vi "Main.vi"(11 "Module Admin":refnum<class "Delacor_lib_QMH_Cloneable Module Admin.lvclass">) -> ()   [LabVIEW 2020, in "My Cloneable Module.lvlib"]
doc: "This template is based off of the Queued Message Handler design pattern and the Queued Message Handler project template that ships with LabVIEW.\n\nThe main difference is that the queue is private to this module and communication between modules is performed via Broadcast and Request events.\n\nRequest events are wrapped in public API methods and are handled in the Event Handling Loop (EHL) of this VI. Any module can register for Broadcast events sent by this module. The EHL generates messages based on user interface actions.\n\nThe Message Handling Loop (MHL) processes messages generated by the EHL, or by other messages. The messages are string values, so new messages can be added easily to the Message Cases case structure in the MHL. Each message cluster can also provide an optional value for Message Data, which is a variant that can be converted to whatever message-specific data is required.\n_____\nBased on Delacor QMH Project Template 5.0.0.82."
uses:
  My Cloneable Module.lvlib
  <vilib>/Delacor/Delacor QMH/Libraries/Cloneable Module Admin_class/Delacor_lib_QMH_Cloneable Module Admin.lvclass
  C:/Program Files (x86)/National Instruments/LabVIEW 2020/vi.lib/Delacor/Delacor QMH/Libraries/Module Admin_class/Delacor_lib_QMH_Module Admin.lvclass
  Module Data--cluster.ctl
  Do Something Argument--cluster.ctl
  <vilib>/Delacor/Delacor QMH/Libraries/Cloneable Module Admin_class/Delacor_lib_QMH_Cloneable Module Admin.lvclass/Delacor_lib_QMH_Cloneable Module Admin.ctl
  <vilib>/Delacor/Delacor QMH/Libraries/Message Queue_class/Delacor_lib_QMH_Message Queue.lvclass/Delacor_lib_QMH_Message Queue.ctl
  Do Something Else Argument--cluster.ctl
  Do Something Else and Wait for Reply Argument--cluster.ctl
  Do Something Else and Wait (Reply Payload)--cluster.ctl
  Stop Argument--cluster.ctl
  <vilib>/Delacor/Delacor QMH/Libraries/Module Admin_class/Delacor_lib_QMH_Module Admin.lvclass/Delacor_lib_QMH_Module Admin.ctl
  <vilib>/Utility/miscctls.llb/LVPointTypeDef.ctl
  <vilib>/Delacor/Delacor QMH/Libraries/Message Queue_class/Delacor_lib_QMH_Enqueue Message (Single).vi
  <vilib>/Delacor/Delacor QMH/Libraries/Cloneable Module Admin_class/Delacor_lib_QMH_Get Module ID.vi
  <vilib>/Delacor/Delacor QMH/Libraries/Module Admin_class/Delacor_lib_QMH_Get External Launch.vi
  <vilib>/Utility/error.llb/Error Cluster From Error Code.vi
  <vilib>/ErrorRing/Error Ring.xnode
  <vilib>/Delacor/Delacor QMH/Libraries/Message Queue_class/Delacor_lib_QMH_Message Queue.lvclass
panel:
  in  "Simulate MHL Error":bool
  in  "Simulate EHL Error":bool
  out "error out":errorcluster
  out "X":dbl
  out "Status":string
  in  "Do Something Else <Replace Me>":bool
  in  "Do Something <Replace Me>":bool
  # "These controls have associated \"Value Changed\" events configured in the Event Structure on the diagram.\n\nReplace them (and reconfigure the Event Structure) with the controls you need for your application. \n\nOther QMH Modules communicate with this Module via its Public API (wrappers for its Request Events).\n\nThis Module communicates with other Modules via its Broadcast Events.\nAny module that wants to get these messages, just registers for this module's Broadcast events."
  # "This template is for the Delacor Modified Queued Message Handler design pattern.\n\nSee the block diagram for more information on how to use this template."
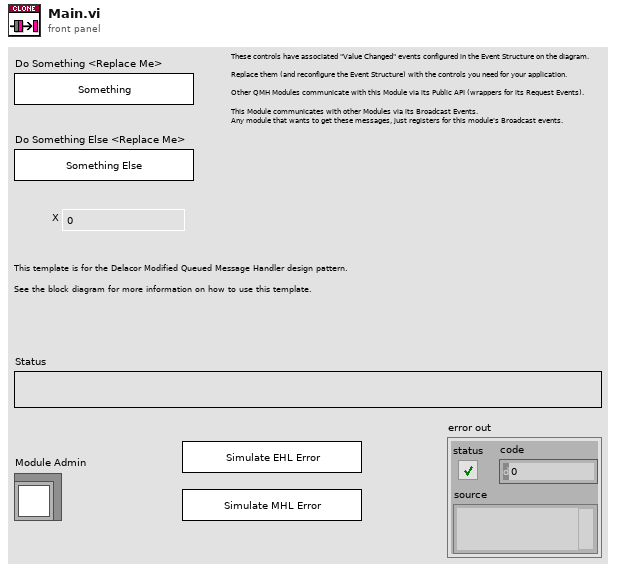
[diagram p1: front panel]
types:
  T1 = typedef "My Cloneable Module.lvlib/Request Events--cluster.ctl" = cluster{"Stop Module":refnum<user-event>, "Do Something":refnum<user-event>, "Do Something Else":refnum<user-event>, "Do Something Else and Wait for Reply":refnum<user-event>, "Show Panel":refnum<user-event>, "Hide Panel":refnum<user-event>, "Show Diagram":refnum<user-event>, "Get Module Execution Status":refnum<user-event>}
  T2 = typedef "My Cloneable Module.lvlib/Module Data--cluster.ctl" = cluster{"Status":string}
  T3 = typedef "My Cloneable Module.lvlib/Do Something Argument--cluster.ctl" = cluster{"Module ID":i32, "Do Something Msg":string}
  T4 = typedef "My Cloneable Module.lvlib/Do Something Else Argument--cluster.ctl" = cluster{"Module ID":i32, "Do Something Else Msg":string, "X":dbl}
  T5 = typedef "My Cloneable Module.lvlib/Do Something Else and Wait for Reply Argument--cluster.ctl" = cluster{"Module ID":i32, "Do Something Else Msg":string, "X":dbl, "Wait Notifier":refnum<notifier>, "wait for reply":bool}
  T6 = enum32{"invalid lock state", "Not Locked", "Locked (No Password)", "Password-protected"}
  T7 = typedef "My Cloneable Module.lvlib/Stop Argument--cluster.ctl" = cluster{"Module ID":i32, "Origin":string, "Exit via Stop Module Req?":bool, "Wait for Module to stop?":bool}
  T8 = typedef "LVPointTypeDef.ctl" = cluster{"Horizontal":i16, "Vertical":i16}
  T9 = enum32{"Invalid", "Standard", "Closed", "Hidden", "Minimized", "Maximized"}
  T10 = typedef "My Cloneable Module.lvlib/Do Something Else and Wait (Reply Payload)--cluster.ctl" = cluster{"Value":dbl, "error":errorcluster}
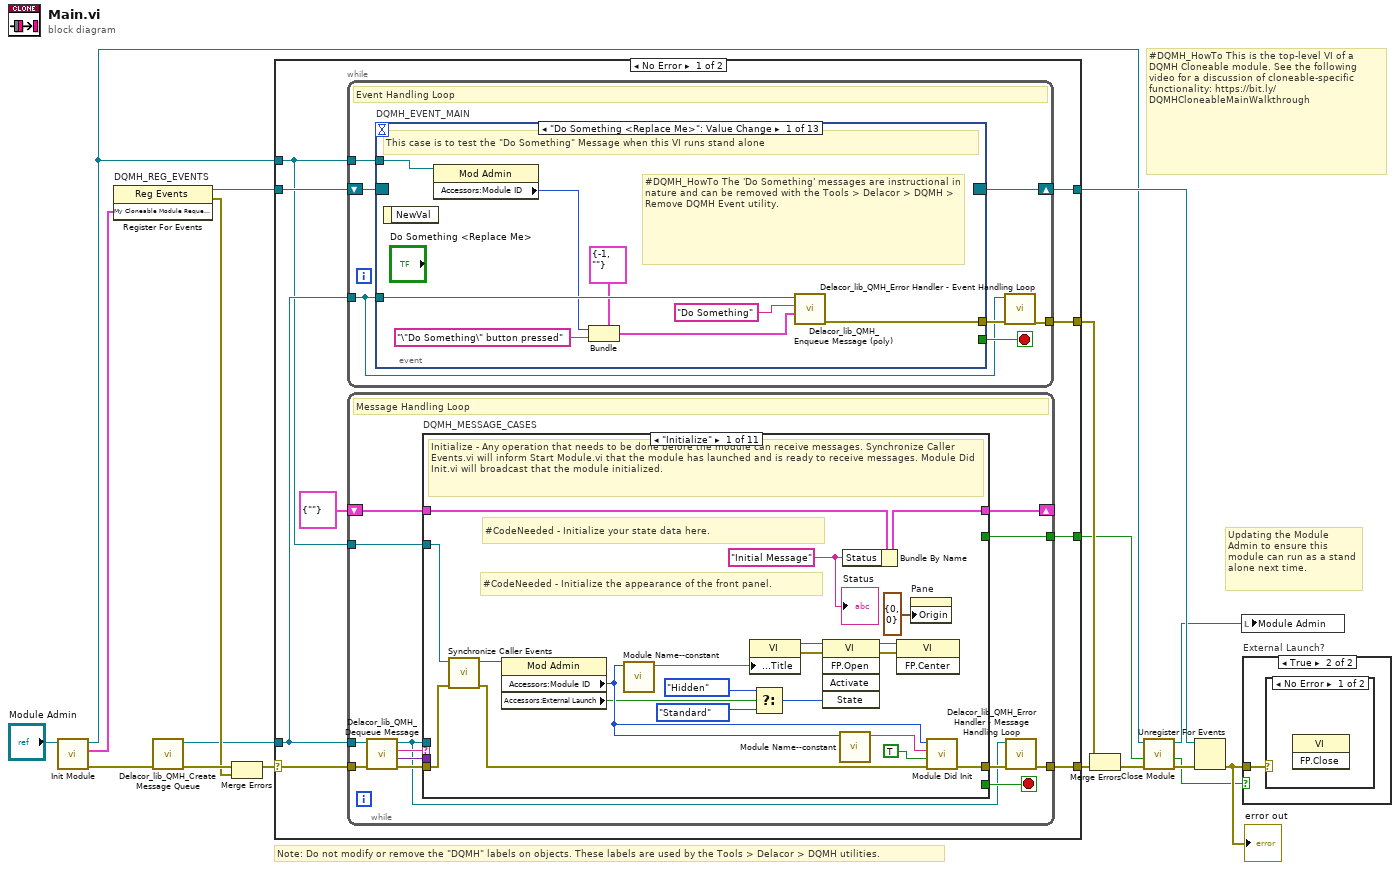
[diagram p0: block diagram]
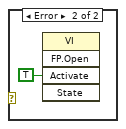
[diagram p3: hidden frame]
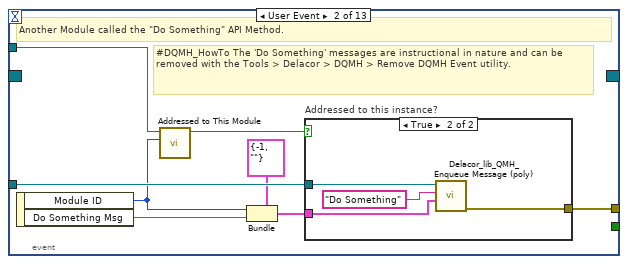
[diagram p4: hidden frame]
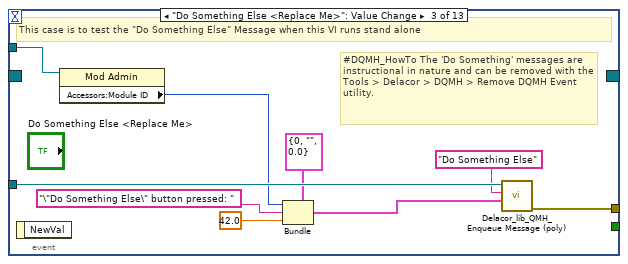
[diagram p6: hidden frame]
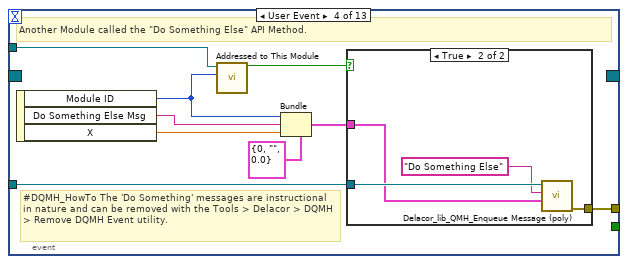
[diagram p7: hidden frame]
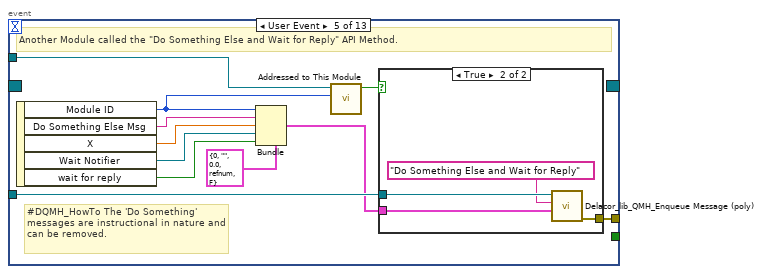
[diagram p9: hidden frame]
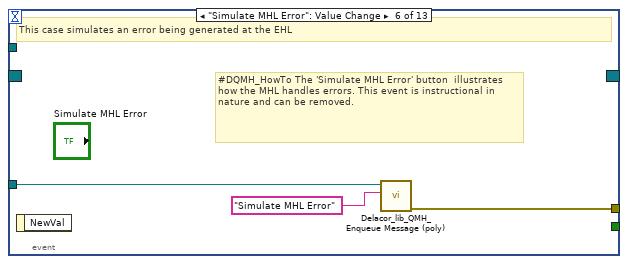
[diagram p11: hidden frame]
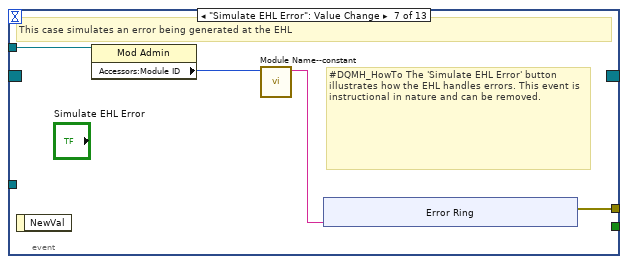
[diagram p12: hidden frame]
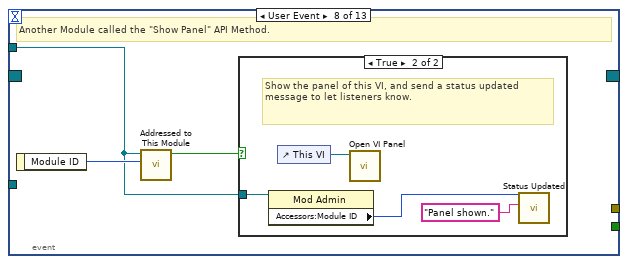
[diagram p13: hidden frame]
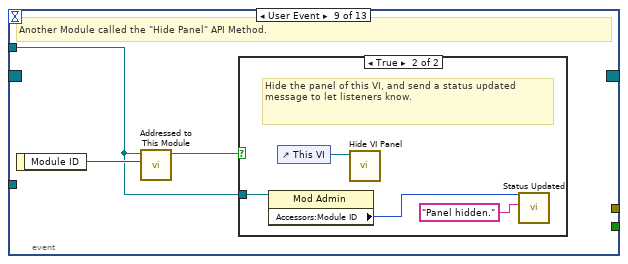
[diagram p15: hidden frame]
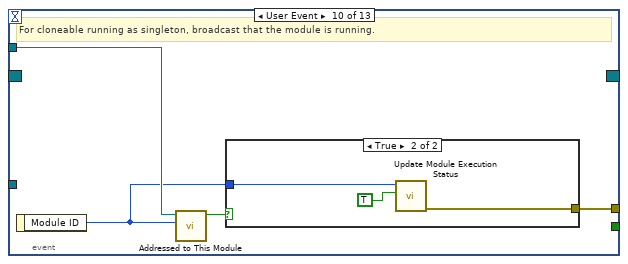
[diagram p17: hidden frame]
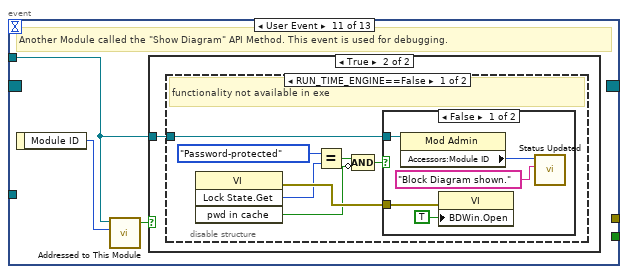
[diagram p19: hidden frame]
diagram:
  # "#DQMH_HowTo This is the top-level VI of a DQMH Cloneable module. See the following video for a discussion of cloneable-specific functionality: https://bit.ly/DQMHCloneableMainWalkthrough"
  # "Note: Do not modify or remove the \"DQMH\" labels on objects. These labels are used by the Tools > Delacor > DQMH utilities."
  # "Updating the Module Admin to ensure this module can run as a stand alone next time."
  n1 = call "Init Module.vi"("Cloneable Module Admin in"="Module Admin") -> ("error out"=w15:errorcluster, "My Cloneable Module Request Events"=w7:T1, "Cloneable Module Admin out"=w4:refnum<class "Delacor_lib_QMH_Cloneable Module Admin.lvclass">)  [unwired: 8 in]
  n2 = register-events "DQMH_REG_EVENTS"(w7) -> (reference out=w8:refnum<event-registration>, error out=w10:errorcluster)  [unwired: 2 in]
  n3 = call <vilib>:"Delacor_lib_QMH_Create Message Queue.vi"("error in (no error)"=w15) -> ("error out"=w12:errorcluster, "Message Queue"=w6:refnum<class "Delacor_lib_QMH_Message Queue.lvclass">)  [unwired: 9 in]
  n4 = Merge Errors(w12, w10) -> (w11:errorcluster)
  n5 = case shown="No Error" w11 {
    selector: w11 -> [w25 w335]
    tunnel: [w27 w334] -> w16
    tunnel: [w24 w342] -> w9
    tunnel: w8 -> [w22 w342]
    tunnel: w6 -> [w21 w333]
    tunnel: [w26 _] -> w17
    tunnel: w4 -> [w20 w338]
    tunnel: [w19 _] -> w2
    frame No Error {
      n6 = while {
        tunnel: w21 -> [w28]
        shift-right: [w31] -> w24
        shift-left: w22 -> [w32]
        tunnel: [w33] -> w26
        tunnel: w20 -> [w29]
        stop <- w30 stop-if-true
        # "Event Handling Loop"
        n7 = event "DQMH_EVENT_MAIN" shown="[0] \"Do Something <Replace Me>\": Value Change" {
          selector: w32 -> [_ _ _ _ _ _ _ _ _ _ _ _ _]
          dyn-events: [_ _ _ _ _ _ _ _ _ _ _ _ _] -> w31
          timeout: _ -> [_ _ _ _ _ _ _ _ _ _ _ _ _]
          tunnel: [_ _ _ _ _ _ _ _ _ _ _ w146 _] -> w30
          tunnel: w28 -> [w41 w49 w62 w71 w86 w93 _ _ _ _ _ w149 w165]
          tunnel: [w42 w50 w63 w72 w87 w94 w98 _ _ w123 _ w150 w168] -> w34
          tunnel: w29 -> [w37 w47 w56 w69 w84 _ w97 w106 w113 w121 w127 w148 w166]
          event "Do Something <Replace Me>": Value Change {
            # "#DQMH_HowTo The 'Do Something' messages are instructional in nature and can be removed with the Tools > Delacor > DQMH > Remove DQMH Event utility."
            # "This case is to test the \"Do Something\" Message when this VI runs stand alone"
            n8 = event-data() -> ()  [unwired: 1 in, 1 out]
            n9 = property class="Mod Admin"(reference=w37) -> ("Accessors:Module ID"=w36:i32)  [unwired: 1 in, 2 out]
            n10 = Bundle(cluster=T3 {"Module ID"=-1, "Do Something Msg"=""} ("Do Something Argument"), "Module ID"=w36, "Do Something Msg"="\"Do Something\" button pressed" ("\"Do Something\" button pressed")) -> (w39:T3)
            n11 = call-poly <vilib>:"Delacor_lib_QMH_Enqueue Message (poly).vi"("Message Data"=w39, "Message"="Do Something", "Message Queue in"=w41) -> ("error out"=w42:errorcluster)  [unwired: 7 in, 1 out]
          }
          event User Event {
            # "#DQMH_HowTo The 'Do Something' messages are instructional in nature and can be removed with the Tools > Delacor > DQMH > Remove DQMH Event utility."
            # "Another Module called the \"Do Something\" API Method."
            n12 = event-data() -> ("Module ID"=w44:i32, "Do Something Msg"=w43:string)  [unwired: 1 in]
            n13 = call "Addressed to This Module.vi"("Module ID from Argument"=w44, "Module Admin"=w47) -> ("Addressed to this instance?"=w48:bool)  [unwired: 8 in, 1 out]
            n14 = Bundle(cluster=T3 {"Module ID"=-1, "Do Something Msg"=""} ("Do Something Argument"), "Module ID"=w44, "Do Something Msg"=w43) -> (w46:T3)
            n15 = case "Addressed to this instance?" shown="True" w48 {
              tunnel: w49 -> [_ w53]
              tunnel: [_ w54] -> w50
              tunnel: w46 -> [_ w51]
              frame False {
                # "Do nothing"
              }
              frame True {
                n16 = call-poly <vilib>:"Delacor_lib_QMH_Enqueue Message (poly).vi"("Message Data"=w51, "Message"="Do Something", "Message Queue in"=w53) -> ("error out"=w54:errorcluster)  [unwired: 7 in, 1 out]
              }
            }
          }
          event "Do Something Else <Replace Me>": Value Change {
            # "#DQMH_HowTo The 'Do Something' messages are instructional in nature and can be removed with the Tools > Delacor > DQMH > Remove DQMH Event utility."
            # "This case is to test the \"Do Something Else\" Message when this VI runs stand alone"
            n17 = event-data() -> ()  [unwired: 1 in, 1 out]
            n18 = property class="Mod Admin"(reference=w56) -> ("Accessors:Module ID"=w55:i32)  [unwired: 1 in, 2 out]
            n19 = Bundle(cluster=T4 {"Module ID"=0, "Do Something Else Msg"="", "X"=0.0} ("Do Something Else Argument"), "Module ID"=w55, "Do Something Else Msg"="\"Do Something Else\" button pressed: " ("\"Do Something Else\" button pressed"), "X"=42.0) -> (w59:T4)
            n20 = call-poly <vilib>:"Delacor_lib_QMH_Enqueue Message (poly).vi"("Message Data"=w59, "Message"="Do Something Else", "Message Queue in"=w62) -> ("error out"=w63:errorcluster)  [unwired: 7 in, 1 out]
          }
          event User Event {
            # "#DQMH_HowTo The 'Do Something' messages are instructional in nature and can be removed with the Tools > Delacor > DQMH > Remove DQMH Event utility."
            # "Another Module called the \"Do Something Else\" API Method."
            n21 = event-data() -> ("Module ID"=w64:i32, "Do Something Else Msg"=w65:string, "X"=w67:dbl)  [unwired: 1 in]
            n22 = call "Addressed to This Module.vi"("Module ID from Argument"=w64, "Module Admin"=w69) -> ("Addressed to this instance?"=w70:bool)  [unwired: 8 in, 1 out]
            n23 = Bundle(cluster=T4 {"Module ID"=0, "Do Something Else Msg"="", "X"=0.0} ("Do Something Else Argument"), "Module ID"=w64, "Do Something Else Msg"=w65, "X"=w67) -> (w66:T4)
            n24 = case shown="True" w70 {
              tunnel: w71 -> [_ w75]
              tunnel: [_ w76] -> w72
              tunnel: w66 -> [_ w73]
              frame False {
              }
              frame True {
                n25 = call-poly <vilib>:"Delacor_lib_QMH_Enqueue Message (poly).vi"("Message Data"=w73, "Message"="Do Something Else", "Message Queue in"=w75) -> ("error out"=w76:errorcluster)  [unwired: 7 in, 1 out]
              }
            }
          }
          event User Event {
            # "#DQMH_HowTo The 'Do Something' messages are instructional in nature and can be removed."
            # "Another Module called the \"Do Something Else and Wait for Reply\" API Method."
            n26 = event-data() -> ("Module ID"=w82:i32, "Do Something Else Msg"=w80:string, "X"=w79:dbl, "Wait Notifier"=w78:refnum<notifier>, "wait for reply"=w77:bool)  [unwired: 1 in]
            n27 = Bundle(cluster=T5 {"Module ID"=0, "Do Something Else Msg"="", "X"=0.0, "Wait Notifier"=refnum, "wait for reply"=FALSE} ("Do Something Else and Wait for Reply Argument"), "Module ID"=w82, "Do Something Else Msg"=w80, "X"=w79, "Wait Notifier"=w78, "wait for reply"=w77) -> (w81:T5)
            n28 = call "Addressed to This Module.vi"("Module ID from Argument"=w82, "Module Admin"=w84) -> ("Addressed to this instance?"=w85:bool)  [unwired: 8 in, 1 out]
            n29 = case shown="True" w85 {
              tunnel: [_ w91] -> w87
              tunnel: w86 -> [_ w90]
              tunnel: w81 -> [_ w88]
              frame False {
              }
              frame True {
                n30 = call-poly <vilib>:"Delacor_lib_QMH_Enqueue Message (poly).vi"("Message Data"=w88, "Message"="Do Something Else and Wait for Reply", "Message Queue in"=w90) -> ("error out"=w91:errorcluster)  [unwired: 7 in, 1 out]
              }
            }
          }
          event "Simulate MHL Error": Value Change {
            # "#DQMH_HowTo The 'Simulate MHL Error' button  illustrates how the MHL handles errors. This event is instructional in nature and can be removed."
            # "This case simulates an error being generated at the EHL"
            n31 = event-data() -> ()  [unwired: 1 in, 1 out]
            n32 = call-poly <vilib>:"Delacor_lib_QMH_Enqueue Message (poly).vi"("Message"="Simulate MHL Error", "Message Queue in"=w93) -> ("error out"=w94:errorcluster)  [unwired: 8 in, 1 out]
          }
          event "Simulate EHL Error": Value Change {
            # "#DQMH_HowTo The 'Simulate EHL Error' button  illustrates how the EHL handles errors. This event is instructional in nature and can be removed."
            # "This case simulates an error being generated at the EHL"
            n33 = event-data() -> ()  [unwired: 1 in, 1 out]
            n34 = property class="Mod Admin"(reference=w97) -> ("Accessors:Module ID"=w96:i32)  [unwired: 1 in, 2 out]
            n35 = call "Module Name--constant.vi"("Module ID"=w96) -> ("Module Name"=w95:string)  [unwired: 10 in]
            n36 = xnode "Error Ring"("parameter 0"=w95) -> ("error out"=w98:errorcluster)
          }
          event User Event {
            # "Another Module called the \"Show Panel\" API Method."
            n37 = event-data() -> ("Module ID"=w107:i32)  [unwired: 1 in]
            n38 = call "Addressed to This Module.vi"("Module ID from Argument"=w107, "Module Admin"=w106) -> ("Addressed to this instance?"=w108:bool)  [unwired: 8 in, 1 out]
            n39 = case shown="True" w108 {
              tunnel: w106 -> [_ w110]
              frame False {
              }
              frame True {
                # "Show the panel of this VI, and send a status updated message to let listeners know."
                n40 = property class="Mod Admin"(reference=w110) -> ("Accessors:Module ID"=w109:i32)  [unwired: 1 in, 2 out]
                n41 = control-ref of="This VI"() -> (w112:refnum<vi>)
                n42 = call "Open VI Panel.vi"("VI"=w112) -> ()  [unwired: 10 in, 1 out]
                n43 = call "Status Updated.vi"("Status"="Panel shown." ("format string"), "Module ID"=w109) -> ()  [unwired: 9 in, 1 out]
              }
            }
          }
          event User Event {
            # "Another Module called the \"Hide Panel\" API Method."
            n44 = event-data() -> ("Module ID"=w114:i32)  [unwired: 1 in]
            n45 = call "Addressed to This Module.vi"("Module ID from Argument"=w114, "Module Admin"=w113) -> ("Addressed to this instance?"=w115:bool)  [unwired: 8 in, 1 out]
            n46 = case shown="True" w115 {
              tunnel: w113 -> [_ w117]
              frame False {
              }
              frame True {
                # "Hide the panel of this VI, and send a status updated message to let listeners know."
                n47 = property class="Mod Admin"(reference=w117) -> ("Accessors:Module ID"=w116:i32)  [unwired: 1 in, 2 out]
                n48 = control-ref of="This VI"() -> (w119:refnum<vi>)
                n49 = call "Hide VI Panel.vi"("VI"=w119) -> ()  [unwired: 10 in, 1 out]
                n50 = call "Status Updated.vi"("Status"="Panel hidden." ("format string"), "Module ID"=w116) -> ()  [unwired: 9 in, 1 out]
              }
            }
          }
          event User Event {
            # "For cloneable running as singleton, broadcast that the module is running."
            n51 = event-data() -> ("Module ID"=w120:i32)  [unwired: 1 in]
            n52 = call "Addressed to This Module.vi"("Module ID from Argument"=w120, "Module Admin"=w121) -> ("Addressed to this instance?"=w122:bool)  [unwired: 8 in, 1 out]
            n53 = case shown="True" w122 {
              tunnel: [_ w126] -> w123
              tunnel: w120 -> [_ w125]
              frame False {
              }
              frame True {
                n54 = call "Update Module Execution Status.vi"("Running?"=TRUE, "Module ID"=w125) -> ("error out"=w126:errorcluster)  [unwired: 9 in]
              }
            }
          }
          event User Event {
            # "Another Module called the \"Show Diagram\" API Method. This event is used for debugging."
            n55 = event-data() -> ("Module ID"=w128:i32)  [unwired: 1 in]
            n56 = call "Addressed to This Module.vi"("Module ID from Argument"=w128, "Module Admin"=w127) -> ("Addressed to this instance?"=w129:bool)  [unwired: 8 in, 1 out]
            n57 = case shown="True" w129 {
              tunnel: w127 -> [_ w130]
              frame False {
              }
              frame True {
                n58 = disable-structure shown="RUN_TIME_ENGINE==False" {
                  disable-tunnel: w130 -> [w131 _]
                  frame condition #0 (active) {
                    # "functionality not available in exe"
                    n59 = invoke class="VI" method="Lock State.Get"() -> (error out=w137:errorcluster, "Get Lock State"=w136:T6, "pwd in cache"=w133:bool)  [unwired: 4 in, 1 out]
                    n60 = Equal?(x=T6."Password-protected", y=w136) -> (x = y?=w134:bool)
                    n61 = Compound Arithmetic op=AND(w134, invert w133) -> (w132:bool)
                    n62 = case shown="False" w132 {
                      tunnel: w137 -> [w142 _]
                      tunnel: w131 -> [w139 _]
                      frame False {
                        n63 = property class="Mod Admin"(reference=w139) -> ("Accessors:Module ID"=w138:i32)  [unwired: 1 in, 2 out]
                        n64 = property class="VI"(error in=w142, "BDWin.Open"=TRUE ("Block Diagram Window:Open")) -> ()  [unwired: 1 in, 2 out]
                        n65 = call "Status Updated.vi"("Status"="Block Diagram shown." ("format string"), "Module ID"=w138) -> ()  [unwired: 9 in, 1 out]
                      }
                      frame True {
                        # "Password-protected VI, and the password is not in the cache. Do not show the diagram."
                      }
                    }
                  }
                  frame condition #1 {
                  }
                }
              }
            }
          }
          event User Event {
            # "Another Module called the \"Stop Module\" API Method  or the Message Handling Loop below."
            n66 = event-data() -> ("Module ID"=w144:i32, "Wait for Module to stop?"=w145:bool, "Origin"=w143:string)  [unwired: 1 in]
            n67 = call "Addressed to This Module.vi"("Module ID from Argument"=w144, "Module Admin"=w148) -> ("Addressed to this instance?"=w147:bool)  [unwired: 8 in, 1 out]
            n68 = case shown="True" w147 {
              tunnel: [_ w162] -> w150
              tunnel: w149 -> [_ w158]
              tunnel: [_ TRUE] -> w146
              tunnel: w145 -> [_ w153]
              tunnel: w144 -> [_ w155]
              tunnel: w143 -> [_ w151]
              frame False {
              }
              frame True {
                # "The event can get fired from the Exit message. The queue gets destroyed there. In this case, the Enqueue VI will return error 1. It is safe to ignore, because the module is already exiting."
                n69 = local write "Status"(w151) -> ()
                n70 = Bundle By Name(cluster=T7 {"Module ID"=-1, "Origin"="", "Exit via Stop Module Req?"=FALSE, "Wait for Module to stop?"=FALSE} ("Stop Argument"), "Module ID"=w155, "Exit via Stop Module Req?"=TRUE, "Wait for Module to stop?"=w153) -> (w152:T7)
                n71 = call-poly <vilib>:"Delacor_lib_QMH_Enqueue Message (poly).vi"("Priority Message? (F)"=TRUE, "Message Data"=w152, "Message"="Exit", "Message Queue in"=w158) -> ("error out"=w163:errorcluster)  [unwired: 6 in, 1 out]
                n72 = call <vilib>:"Clear Errors.vi"("error in (no error)"=w163, "specific error code to clear (0: all)"=1) -> ("error out"=w162:errorcluster)  [unwired: 4 in, 1 out]
              }
            }
          }
          event Panel Close? {
            w167 = TRUE  # Discard the event, the MHL is responsible for closing and stopping this VI.
            # "Hide the panel or send the 'Exit' message if the user clicks the 'X' on the module main VI panel."
            n73 = event-data() -> ()  [unwired: 1 in, 1 out]
            n74 = property class="Mod Admin"(reference=w166) -> ("Accessors:External Launch"=w164:bool)  [unwired: 1 in, 2 out]
            n75 = case shown="True" w164 {
              tunnel: w165 -> [_ w172]
              tunnel: [_ w173] -> w168
              frame True {
                # "If externally launched, clicking the 'X' hides the panel, but doesn't close it."
                n76 = control-ref of="This VI"() -> (w169:refnum<vi>)
                n77 = call "Hide VI Panel.vi"("VI"=w169) -> ()  [unwired: 10 in, 1 out]
              }
              frame False {
                # "If run as a stand-alone VI, clicking the panel 'X' stops the VI."
                n78 = call-poly <vilib>:"Delacor_lib_QMH_Enqueue Message (poly).vi"("Priority Message? (F)"=TRUE, "Message"="Exit", "Message Queue in"=w172) -> ("error out"=w173:errorcluster)  [unwired: 7 in, 1 out]
              }
            }
            n79 = event-data("Discard?"=w167) -> ()  [unwired: 1 in, 1 out]
          }
        }
        n80 = call-dynamic "Delacor_lib_QMH_Error Handler - Event Handling Loop.vi"("error in (no error)"=w34, "Message Queue in"=w28) -> ("dup error in"=w33:errorcluster)  [unwired: 8 in, 1 out]
      }
      n81 = while {
        tunnel: w21 -> [w177]
        shift-right: [w181] -> _
        shift-left: T2 {"Status"=""} ("Data Cluster") -> [w182]
        tunnel: w25 -> [w185]
        tunnel: [w183] -> w27
        tunnel: w20 -> [w175]
        tunnel: [w174] -> w19
        stop <- w180 stop-if-true
        # "Message Handling Loop"
        n82 = call-dynamic "Delacor_lib_QMH_Dequeue Message.vi"("error in (no error)"=w185, "Message Queue in"=w177) -> ("error out"=w184:errorcluster, "Message Data"=w178:variant, "Message"=w179:string, "Message Queue out"=w176:refnum<class "Delacor_lib_QMH_Message Queue.lvclass">)  [unwired: 6 in]
        n83 = case "DQMH_MESSAGE_CASES" shown="\"Initialize\"" w179 {
          selector: w179 -> [_ _ _ _ _ _ _ _ _ _ w320]
          tunnel: w176 -> [_ _ _ _ _ _ _ w271 _ w310 _]
          tunnel: w184 -> [w205 w209 w219 w230 w251 w266 w268 w280 w293 w316 w322]
          tunnel: [w203 w209 w217 w229 w250 w265 w268 w276 w292 w313 w323] -> w186
          tunnel: w182 -> [w196 w208 w216 w228 w248 w264 w267 w275 w290 w309 w321]
          tunnel: [w195 w208 w216 w228 w248 w264 w267 w275 w290 w309 w321] -> w181
          tunnel: [_ _ _ _ _ _ _ _ _ w308 _] -> w180
          tunnel: w178 -> [_ _ w215 w225 w245 _ _ w274 _ w306 _]
          tunnel: w175 -> [w190 _ w211 w221 w235 _ _ w273 w288 w302 w318]
          tunnel: [_ _ _ _ _ _ _ _ _ w304 _] -> w174
          frame "Initialize" {
            w187 = "Initial Message" ("Initial Message")
            # "#CodeNeeded - Initialize the appearance of the front panel."
            # "#CodeNeeded - Initialize your state data here."
            # "Initialize - Any operation that needs to be done before the module can receive messages. Synchronize Caller Events.vi will inform Start Module.vi that the module has launched and is ready to receive messages. Module Did Init.vi will broadcast that the module initialized."
            n84 = call "Synchronize Caller Events.vi"("error in (no error)"=w205, "Module Admin"=w190) -> ("error out"=w204:errorcluster, "Module Admin out"=w189:refnum<class "Delacor_lib_QMH_Cloneable Module Admin.lvclass">)  [unwired: 8 in]
            n85 = property class="Mod Admin"(reference=w189) -> ("Accessors:Module ID"=w192:i32, "Accessors:External Launch"=w191:bool)  [unwired: 1 in, 2 out]
            n86 = call "Module Name--constant.vi"("Module ID"=w192) -> ("Module Name"=w200:string)  [unwired: 10 in]
            n87 = property class="VI"("Front Panel.Title"=w200) -> (reference out=w202:refnum<vi>, error out=w207:errorcluster)  [unwired: 2 in]
            n88 = Select(t=T9."Hidden" ("State"), s=w191, f=T9."Standard" ("State")) -> (s? t:f=w197:T9)
            n89 = invoke class="VI" method="FP.Open"(reference=w202, error in=w207, "State"=w197) -> (reference out=w201:refnum<vi>, error out=w206:errorcluster)  [unwired: 2 in, 3 out]
            n90 = call "Module Name--constant.vi"("Module ID"=w192) -> ("Module Name"=w193:string)  [unwired: 10 in]
            n91 = Bundle By Name(cluster=w196, "Status"=w187) -> (w195:T2)
            n92 = invoke class="VI" method="FP.Center"(reference=w201, error in=w206) -> ()  [unwired: 1 in, 3 out]
            n93 = property on="Pane" class="Pane"("Origin"=T8 {"Horizontal"=0, "Vertical"=0}) -> ()  [unwired: 2 in, 2 out]
            n94 = call "Module Did Init.vi"("error in (no error)"=w204, "Initialized?"=TRUE, "Origin"=w193, "Module ID"=w192) -> ("error out"=w203:errorcluster)  [unwired: 7 in]
            "Status" <- w187
          }
          frame "--- Module Specific ---" {
            # "Separator -- The following cases handle messages specific to this Module."
          }
          frame "Do Something" {
            # "#DQMH_HowTo The 'Do Something' messages are instructional in nature and can be removed with the Tools > Delacor > DQMH > Remove DQMH Event utility."
            # "Do Something - Replace this message with functionality for your own application. Note that this message also fires the \"Did Something\" broadcast event."
            n95 = property class="Mod Admin"(reference=w211) -> ("Accessors:Module ID"=w210:i32)  [unwired: 1 in, 2 out]
            n96 = Variant To Data(error in=w219, type=T3 {"Module ID"=-1, "Do Something Msg"=""} ("Do Something Argument"), Variant=w215) -> (data=w214:T3, error out=w218:errorcluster)
            n97 = Unbundle By Name(w214) -> ("Do Something Msg"=w212:string)
            n98 = call "Status Updated.vi"("Status"=w212, "Module ID"=w210) -> ()  [unwired: 9 in, 1 out]
            n99 = local write "Status"(w212) -> ()
            n100 = call "Did Something.vi"("error in (no error)"=w218, "Did Something Msg"=w212, "Module ID"=w210) -> ("error out"=w217:errorcluster)  [unwired: 8 in]
          }
          frame "Do Something Else" {
            # "#DQMH_HowTo The 'Do Something' messages are instructional in nature and can be removed with the Tools > Delacor > DQMH > Remove DQMH Event utility."
            # "Do Something Else - Replace this message with functionality for your own application."
            n101 = Variant To Data(error in=w230, type=T4 {"Module ID"=0, "Do Something Else Msg"="", "X"=0.0} ("Do Something Else Argument"), Variant=w225) -> (data=w226:T4, error out=w229:errorcluster)
            n102 = Unbundle By Name(w226) -> ("Do Something Else Msg"=w224:string, "X"=w223:dbl)
            "X" <- w223
            n103 = property class="Mod Admin"(reference=w221) -> ("Accessors:Module ID"=w220:i32)  [unwired: 1 in, 2 out]
            n104 = Format Into String(initial string=w224, w223) -> (resulting string=w222:string)  [unwired: 2 in, 1 out]
            n105 = call "Status Updated.vi"("Status"=w222, "Module ID"=w220) -> ()  [unwired: 9 in, 1 out]
            n106 = local write "Status"(w222) -> ()
          }
          frame "Do Something Else and Wait for Reply" {
            w238 = "X(%.2f)+Offset(%.2f)=%.2f"  # status message format string
            # "#DQMH_HowTo The 'Do Something' messages are instructional in nature and can be removed."
            # "Send back X with a random offset"
            # "Do Something Else and Wait for Reply - Replace this message with functionality for your own application. Note that this message must fire a notifier to let callers know it has finished execution, and it returns an error if the 'Value' is negative."
            n107 = Variant To Data(error in=w251, type=T5 {"Module ID"=0, "Do Something Else Msg"="", "X"=0.0, "Wait Notifier"=refnum, "wait for reply"=FALSE} ("Do Something Else and Wait for Reply Argument"), Variant=w245) -> (data=w246:T5, error out=w232:errorcluster)
            n108 = Unbundle By Name(w246) -> ("Wait Notifier"=w243:refnum<notifier>, "Do Something Else Msg"=w244:string, "X"=w240:dbl, "wait for reply"=w231:bool)
            n109 = property class="Mod Admin"(reference=w235) -> ("Accessors:Module ID"=w234:i32)  [unwired: 1 in, 2 out]
            n110 = Random Number (0-1)() -> (number: 0 to 1=w239:dbl)
            n111 = local write "X"(w240) -> ()
            n112 = Add(x=w239, y=w240) -> (x+y=w233:dbl)
            n113 = Format Into String(format string=w238, initial string=w244, w240, w239, w233) -> (resulting string=w236:string)  [unwired: 1 in, 1 out]
            n114 = Less Than 0?(x=w233) -> (x < 0?=w237:bool)
            n115 = case shown="True" w237 {
              tunnel: [_ w258] -> w249
              frame False {
              }
              frame True {
                n116 = xnode "Error Ring"() -> ("error out"=w258:errorcluster)
              }
            }
            n117 = Bundle By Name(cluster=T10 {"Value"=0.0, "error"={"status"=FALSE, "code"=0, "source"=""}} ("notification"), "error"=w249, "Value"=w233) -> (w241:T10)
            n118 = local write "Status"(w236) -> ()
            n119 = call "Status Updated.vi"("Status"=w236, "Module ID"=w234) -> ()  [unwired: 9 in, 1 out]
            n120 = case shown="True" w231 {
              tunnel: w243 -> [_ w255]
              tunnel: w241 -> [_ w254]
              frame False {
              }
              frame True {
                # "Simulate an operation that requires a wait."
                n121 = Wait (ms)(milliseconds to wait=u32 1000) -> (millisecond timer value=w252:u32)
                n122 = flat-sequence {
                  tunnel: w255 -> [w257]
                  tunnel: w254 -> [w256]
                  tunnel: w252 -> [_]
                  frame #0 {
                    n123 = Send Notification(notification=w256, notifier=w257) -> ()  [unwired: 1 in, 2 out]
                  }
                }
              }
            }
            n124 = Merge Errors(w232, w249) -> (w250:errorcluster)
          }
          frame "---Copy This Frame---" {
            # "Duplicate this frame when creating new messages.  Change this comment in the duplicated frame to describe this message."
            n125 = Merge Errors(w266) -> (w265:errorcluster)
          }
          frame "--- Exit and Error Handling---" {
            # "Separator - the following cases handle errors and exit messages."
          }
          frame "Error" {
            # "#CodeRecommended - If you ever change the name of this \"Error\" message, you'll need to update the name in the Check Loop Error.vi as well."
            # "#CodeRecommended - If the module is running in standalone mode (External Launch = FALSE), this code will pop up an error dialog and call the 'Exit' message if an error occurs. Add more fine-grained error handling here."
            # "Error - Check the error message data and respond accordingly. This message is sent by the \"Error Handler\" VIs at the end of each loop in this application."
            n126 = property class="Mod Admin"(reference=w273) -> ("Accessors:External Launch"=w272:bool, "Accessors:Module ID"=w269:i32)  [unwired: 1 in, 2 out]
            n127 = Variant To Data(error in=w280, type=errorcluster {"status"=FALSE, "code"=0, "source"=""} ("error constant"), Variant=w274) -> (data=w281:errorcluster, error out=w278:errorcluster)
            n128 = call "Module Name--constant.vi"("Module ID"=w269) -> ("Module Name"=w270:string)  [unwired: 10 in]
            n129 = call "Error Reported.vi"("Additional Information"=w270, "Error"=w281, "Module ID"=w269) -> ()  [unwired: 8 in, 1 out]
            n130 = case shown="False" w272 {
              tunnel: [w286 _] -> w277
              tunnel: w271 -> [w284 _]
              tunnel: w281 -> [w285 _]
              frame False {
                # "If the module is running standalone, then pop up an error dialog and call the \"Exit\" message."
                n131 = call <vilib>:"Simple Error Handler.vi"("error in (no error)"=w285) -> ()  [unwired: 4 in, 5 out]
                n132 = call-poly <vilib>:"Delacor_lib_QMH_Enqueue Message (poly).vi"("Priority Message? (F)"=TRUE, "Message"="Exit", "Message Queue in"=w284) -> ("error out"=w286:errorcluster)  [unwired: 7 in, 1 out]
              }
              frame True {
                # "If the module was launched externally, calling the Error Reported broadcast VI is the only action performed by the \"Error\" message. The module's caller can then process the error appropriately."
              }
            }
            n133 = Merge Errors(w278, w277) -> (w276:errorcluster)
            n134 = local write "error out"(w276) -> ()
          }
          frame "Simulate MHL Error" {
            # "#DQMH_HowTo The 'Simulate MHL Error' button  illustrates how the MHL handles errors. This event is instructional in nature and can be removed."
            # "Simulate an error occurring at the MHL"
            n135 = property class="Mod Admin"(reference=w288) -> ("Accessors:Module ID"=w289:i32)  [unwired: 1 in, 2 out]
            n136 = call "Module Name--constant.vi"("Module ID"=w289) -> ("Module Name"=w287:string)  [unwired: 10 in]
            n137 = xnode "Error Ring"("parameter 0"=w287) -> ("error out"=w291:errorcluster)
            n138 = Merge Errors(w293, w291) -> (w292:errorcluster)
          }
          frame "Exit" {
            w307 = 91  # 91: not all Exit messages will have an argument
            w308 = TRUE  # Stop the VI
            # "Release the message queue reference"
            # "#CodeNeeded - Add any required cleanup code here."
            # "Exit - Exit the application."
            n139 = Variant To Data(error in=w316, type=T7 {"Module ID"=-1, "Origin"="", "Exit via Stop Module Req?"=FALSE, "Wait for Module to stop?"=FALSE} ("Stop Argument"), Variant=w306) -> (data=w303:T7, error out=w311:errorcluster)
            n140 = call <vilib>:"Clear Errors.vi"("error in (no error)"=w311, "specific error code to clear (0: all)"=w307) -> ("error out"=w315:errorcluster)  [unwired: 4 in, 1 out]
            n141 = control-ref of="This VI"() -> (w301:refnum<vi>)
            n142 = call-dynamic "Delacor_lib_QMH_Release Message Queue.vi"("error in (no error)"=w315, "Message Queue"=w310) -> ("error out"=w314:errorcluster)  [unwired: 9 in]
            n143 = call "Handle Exit.vi"("Stop Argument"=w303, "Module Admin in"=w302, "VI reference"=w301) -> ("error out"=w312:errorcluster, "Wait for Stop?"=w304:bool)  [unwired: 7 in]
            n144 = Merge Errors(w314, w312) -> (w313:errorcluster)
          }
          frame Default {
            # "'Default' case only runs if there is a message that isn't defined in any of the other cases.  Output a programming error."
            n145 = property class="Mod Admin"(reference=w318) -> ("Accessors:Module ID"=w317:i32)  [unwired: 1 in, 2 out]
            n146 = call "Module Name--constant.vi"("Module ID"=w317) -> ("Module Name"=w319:string)  [unwired: 10 in]
            n147 = xnode "Error Ring"("parameter 0"=w320, "parameter 1"=w319) -> ("error out"=w324:errorcluster)
            n148 = Merge Errors(w322, w324) -> (w323:errorcluster)
          }
        }
        n149 = call-dynamic "Delacor_lib_QMH_Error Handler - Message Handling Loop.vi"("error in (no error)"=w186, "Message Queue in"=w176) -> ("dup error in"=w183:errorcluster)  [unwired: 8 in, 1 out]
      }
    }
    frame Error {
      n150 = call "Synchronize Caller Events.vi"("Module Admin"=w338) -> ("Module Admin out"=w337:refnum<class "Delacor_lib_QMH_Cloneable Module Admin.lvclass">)  [unwired: 9 in, 1 out]
      n151 = property class="Mod Admin"(reference=w337) -> ("Accessors:Module ID"=w336:i32)  [unwired: 1 in, 2 out]
      n152 = call-dynamic "Delacor_lib_QMH_Release Message Queue.vi"("error in (no error)"=w335, "Message Queue"=w333) -> ("error out"=w334:errorcluster)  [unwired: 9 in]
      n153 = call "Module Name--constant.vi"("Module ID"=w336) -> ("Module Name"=w341:string)  [unwired: 10 in]
      n154 = Format Into String(format string="An error occurred during initialization. %s is no longer running.", w341) -> (resulting string=w339:string)  [unwired: 2 in, 1 out]
      n155 = call "Error Reported.vi"("Additional Information"=w339, "Error"=w334, "Module ID"=w336) -> ()  [unwired: 8 in, 1 out]
    }
  }
  n156 = Merge Errors(w17, w16) -> (w18:errorcluster)
  n157 = call "Close Module.vi"("error in"=w18, "Wait for stop?"=w2, "Module Admin in"=w4) -> ("error out"=w14:errorcluster, "External Launch"=w1:bool, "Module Admin out"=w3:refnum<class "Delacor_lib_QMH_Cloneable Module Admin.lvclass">)  [unwired: 6 in]
  n158 = Unregister For Events(event registration refnum=w9, error in=w14) -> (error out=w13:errorcluster)
  "error out" <- w13
  n159 = local write "Module Admin"(w3) -> ()
  n160 = case "External Launch?" shown="True" w1 {
    tunnel: w13 -> [_ w343]
    frame False {
    }
    frame True {
      n161 = case shown="No Error" w343 {
        frame No Error {
          n162 = invoke class="VI" method="FP.Close"() -> ()  [unwired: 3 in, 3 out]
        }
        frame Error {
          n163 = invoke class="VI" method="FP.Open"("Activate"=TRUE ("Activate?")) -> ()  [unwired: 4 in, 5 out]
        }
      }
    }
  }
